vi "Add DTC.vi"(8 "error in (no error)":errorcluster, 11 "Node Ptr":u64 format="%.0x") -> (0 "error out":errorcluster)   [LabVIEW 2015, in "J1939 Addon System Explorer.lvlib"]
uses:
  J1939 Addon System Explorer.lvlib
  Shared/SubVIs/Constants.vi
  Shared/J1939 Addon Shared.lvlib
  <vilib>/NI VeriStand/Custom Device API/Custom Device API.lvlib
panel:
  in  "Tag":string
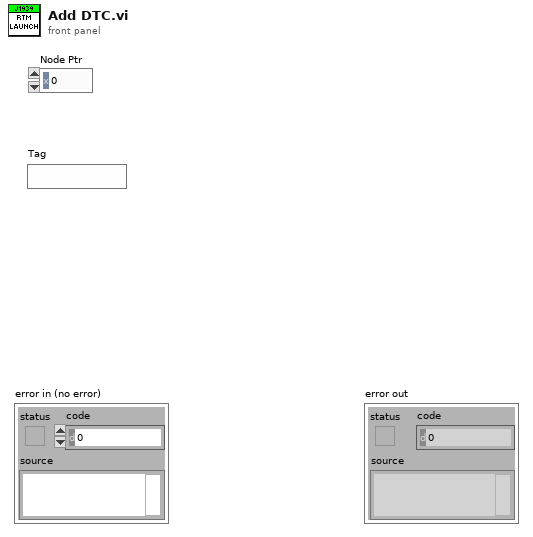
[diagram p1: front panel]
types:
  T1 = typedef "Custom Device API.lvlib/Custom Device Item Ref.ctl" = u64
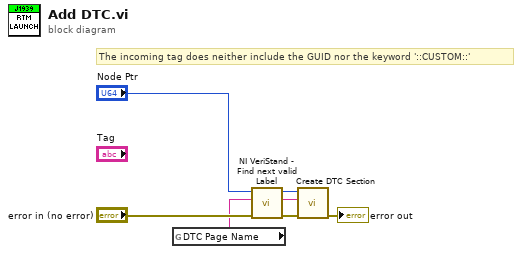
[diagram p0: block diagram]
diagram:
  # "The incoming tag does neither include the GUID nor the keyword '::CUSTOM::'"
  n1 = global read "Constants.vi" "DTC Page Name"() -> (w3:string)
  n2 = call <vilib>:"NI VeriStand - Find next valid Label.vi"("error in (no error)"="error in (no error)", "Label"=w3, "Item Ref in"="Node Ptr") -> ("error out"=w4:errorcluster, "Label out"=w2:string, "Item Ref out"=w6:T1)  [unwired: 4 in, 2 out]
  n3 = call "Create DTC Section.vi"("error in (no error)"=w4, "Name"=w2, "Item Ref in"=w6) -> ("error out"=→"error out":errorcluster)  [unwired: 8 in]
